vi "Serial Table Lookup.vi"(8 "error in (no error)":errorcluster, 9 "Target Serial#:":u32 caption="Serial#:" max=268435455, 10 "Data IN":T1={"Message"="", "Homed?"=FALSE, "NextState"=enum."Timeout", "G.Load"=0.0, "G.Position"=0.0, "Load#"=0, "[G.Loads]"=[], "[TotalLoads]"=[], "[Errors]"=[], "ZeroWait"=0, "Results"=[], "DwellWait"=FALSE, "Test Result"=FALSE, "[CondyleLoads]"=[], "[Max]"=[], "[Min]"=[], "Valid String?"=FALSE, "ScanTime"=timestamp(0 s since 1904-01-01), "ScannedString"="", "LabelDevID"=0, "MfgDate"=timestamp(0 s since 1904-01-01), "[EEPROM Cmds]"=[], "[CalData]"=[], "[A/Ds]"=[], "[A/Dmax]"=[], "[A/Dmin]"=[], "BattMax"=0.0, "BattMin"=0.0, "DwellTime"=2000, "PendingDeviceType"="", "Zero G.load"=0.0, "GAINC Value"="", "Programming Step"=enum."Load EEPROM", "Front Panel Program?"=FALSE, "Final Program?"=FALSE, "PCB Score"=100, "AssyScore"=100, "Pass/Fail #"="", "Result String"="", "Programming Mode"=enum."Initial Program", "Angle Test Step"=enum."Initialize", "Accel Values"=[], "Shutdown Counter"=0, "V1"=0, "V2"=0, "V3"=0, "V4"=0, "EEPROM Data"=[], "Counter"=0, "Page#"=0, "Timer"=timestamp(0 s since 1904-01-01), "Use Mark10?"=FALSE, "Eng-Result#"=0, "DUT Serial #"=0, "Scroll Message?"=FALSE, "Clear Message"=FALSE, "Batt Test Step "=enum."Initialize", "RXTX Window Found?"=FALSE, "Shutdown First Call?"=FALSE, "A2 Delay (msec)"=500, "Support Script"={"Script #"="", "Script Revision"="", "[OEMs]"=[], "[[DeviceTypes]]"=[], "[[DeviceTypesVals]]"=[], "[[List of Errors]]"=[], "Default GAINC"="", "[[ASICtrims]]"=[], "ID For Echo"="", "Condyle A CalFactor"=100, "Condyle B CalFactor"=100, "[OEMs Prefix]"=[], "Packet ID 18"="", "[[Force Table Load Test]]"=[], "[[Force Table AccurTest]]"=[]}, "Serial Table"={"Serial File Path"=path "", "[[Serial Lookup Table]]"=[], "Serial Device Info"=[], "Valid Serial?"=FALSE}, "Target Information"={"Target Brand"="", "Target DeviceType"="", "Target Serial#"=100, "Target Lot#"=0, "Target DevID"=0, "Target Channel"=5}, "Operator"="", "COM Port"="", "Config Path"=path "", "Tx Array"=[], "DUT Parameters"={"Channel"=0, "DeviceID"=0, "Script Rev"=0, "Month"=0, "Day"=0, "Year"=0, "Lot#"=0, "V1"=0, "V2"=0, "V3"=0, "V4"=0, "MFG"=0, "Cal FactorA 10"=0, "Cal FactorB 10  "=0, "Cal FactorA 16"=0, "Cal FactorB 16"=0, "ASICtrim"=[], "TmpChan"=0, "GAINC"="", "Brand"="", "Device"="", "Serial #"=0, "Batt310"=0, "Batt 280"=0}, "FTS Main?"=FALSE, "Loading"={"[Forces]"=[], "[Dwell]"=[], "Loading Step"=enum."Initialize Test"}, "Software Version"="", "Correction Factor"="", "Second Load Test"=FALSE, "Acc Loads"=[], "Mark10 Config"={"H2S%"=[80.0, 85.0, 90.0, 95.0, 100.0], "H2S Speed"=[12.0, 8.0, 6.0, 4.0, 2.0], "H to S"=2.0, "Home Speed"=1.0, "LoadWin"=0.0, "Load Speed"=0.0, "PID"={"Kp"=0.04, "Kd"=0.005001, "Ki"=2.9999999999999923e-05}}, "Channels"={"Transceiver Ch"=5, "Operating Ch"=5, "Start Ch"=0}, "Channel EEPROM"=[], "Load Notes"=[], "Engr Log?"=FALSE, "Time"=[], "Program Retry"=FALSE, "Operator Channel"="", "Target Channel "="", "New Data Program"=FALSE, "NFHU Pass?"=FALSE, "Cycle Number"=0, "Cal Cycle#"=0, "[Avg G.Loads] "=[], "[Avg A/Ds] "=[], "Cal Retry?"=FALSE, "[Total A/Ds]  "=[], "Cycle Num LA"=0, "LA Cycle# "=0, "Shim Num"=0, "Shim#  "=0, "Angle Test?"=FALSE} {"Mark10 Config"."PID"."Ki" min=0.0 max=200.0 format="%.6f"; "Mark10 Config"."PID"."Kd" min=0.0 max=200.0 format="%.6f"; "Mark10 Config"."PID"."Kp" min=0.0 max=200.0 format="%.6f"; "DUT Parameters"."ASICtrim" format="%02x"}) -> (0 "error out":errorcluster, 2 "Valid Serial":bool, 3 "State-machine Local Variables out":T1={"Message"="", "Homed?"=FALSE, "NextState"=enum."Timeout", "G.Load"=0.0, "G.Position"=0.0, "Load#"=0, "[G.Loads]"=[], "[TotalLoads]"=[], "[Errors]"=[], "ZeroWait"=0, "Results"=[], "DwellWait"=FALSE, "Test Result"=FALSE, "[CondyleLoads]"=[], "[Max]"=[], "[Min]"=[], "Valid String?"=FALSE, "ScanTime"=timestamp(0 s since 1904-01-01), "ScannedString"="", "LabelDevID"=0, "MfgDate"=timestamp(0 s since 1904-01-01), "[EEPROM Cmds]"=[], "[CalData]"=[], "[A/Ds]"=[], "[A/Dmax]"=[], "[A/Dmin]"=[], "BattMax"=0.0, "BattMin"=0.0, "DwellTime"=2000, "PendingDeviceType"="", "Zero G.load"=0.0, "GAINC Value"="", "Programming Step"=enum."Load EEPROM", "Front Panel Program?"=FALSE, "Final Program?"=FALSE, "PCB Score"=100, "AssyScore"=100, "Pass/Fail #"="", "Result String"="", "Programming Mode"=enum."Initial Program", "Angle Test Step"=enum."Initialize", "Accel Values"=[], "Shutdown Counter"=0, "V1"=0, "V2"=0, "V3"=0, "V4"=0, "EEPROM Data"=[], "Counter"=0, "Page#"=0, "Timer"=timestamp(0 s since 1904-01-01), "Use Mark10?"=FALSE, "Eng-Result#"=0, "DUT Serial #"=0, "Scroll Message?"=FALSE, "Clear Message"=FALSE, "Batt Test Step "=enum."Initialize", "RXTX Window Found?"=FALSE, "Shutdown First Call?"=FALSE, "A2 Delay (msec)"=500, "Support Script"={"Script #"="", "Script Revision"="", "[OEMs]"=[], "[[DeviceTypes]]"=[], "[[DeviceTypesVals]]"=[], "[[List of Errors]]"=[], "Default GAINC"="", "[[ASICtrims]]"=[], "ID For Echo"="", "Condyle A CalFactor"=100, "Condyle B CalFactor"=100, "[OEMs Prefix]"=[], "Packet ID 18"="", "[[Force Table Load Test]]"=[], "[[Force Table AccurTest]]"=[]}, "Serial Table"={"Serial File Path"=path "", "[[Serial Lookup Table]]"=[], "Serial Device Info"=[], "Valid Serial?"=FALSE}, "Target Information"={"Target Brand"="", "Target DeviceType"="", "Target Serial#"=100, "Target Lot#"=0, "Target DevID"=0, "Target Channel"=5}, "Operator"="", "COM Port"="", "Config Path"=path "", "Tx Array"=[], "DUT Parameters"={"Channel"=0, "DeviceID"=0, "Script Rev"=0, "Month"=0, "Day"=0, "Year"=0, "Lot#"=0, "V1"=0, "V2"=0, "V3"=0, "V4"=0, "MFG"=0, "Cal FactorA 10"=0, "Cal FactorB 10  "=0, "Cal FactorA 16"=0, "Cal FactorB 16"=0, "ASICtrim"=[], "TmpChan"=0, "GAINC"="", "Brand"="", "Device"="", "Serial #"=0, "Batt310"=0, "Batt 280"=0}, "FTS Main?"=FALSE, "Loading"={"[Forces]"=[], "[Dwell]"=[], "Loading Step"=enum."Initialize Test"}, "Software Version"="", "Correction Factor"="", "Second Load Test"=FALSE, "Acc Loads"=[], "Mark10 Config"={"H2S%"=[80.0, 85.0, 90.0, 95.0, 100.0], "H2S Speed"=[12.0, 8.0, 6.0, 4.0, 2.0], "H to S"=2.0, "Home Speed"=1.0, "LoadWin"=0.0, "Load Speed"=0.0, "PID"={"Kp"=0.04, "Kd"=0.005001, "Ki"=2.9999999999999923e-05}}, "Channels"={"Transceiver Ch"=5, "Operating Ch"=5, "Start Ch"=0}, "Channel EEPROM"=[], "Load Notes"=[], "Engr Log?"=FALSE, "Time"=[], "Program Retry"=FALSE, "Operator Channel"="", "Target Channel "="", "New Data Program"=FALSE, "NFHU Pass?"=FALSE, "Cycle Number"=0, "Cal Cycle#"=0, "[Avg G.Loads] "=[], "[Avg A/Ds] "=[], "Cal Retry?"=FALSE, "[Total A/Ds]  "=[], "Cycle Num LA"=0, "LA Cycle# "=0, "Shim Num"=0, "Shim#  "=0, "Angle Test?"=FALSE} {"Mark10 Config"."PID"."Ki" min=0.0 max=200.0 format="%.6f"; "Mark10 Config"."PID"."Kd" min=0.0 max=200.0 format="%.6f"; "Mark10 Config"."PID"."Kp" min=0.0 max=200.0 format="%.6f"; "DUT Parameters"."ASICtrim" format="%02x"})   [LabVIEW 2015]
uses:
  Controls/LocalVars.ctl
  Controls/Gen2 FT states.ctl
  Controls/Iniial Device Programming.ctl
  ProgramStageControl.ctl
  Controls/Batt Cap Steps.ctl
  Controls/Support Script.ctl
  Controls/Serial Table.ctl
  Controls/Device Information.ctl
  Controls/InfoPacket.ctl
  Controls/Loading.ctl
  Controls/Load Step.ctl
  Controls/Mark10 Config.ctl
  Controls/PID parameters.ctl
  Controls/Channels.ctl
panel:
  out "[[DeviceTypesVals]]":u16[][](array[numeric])
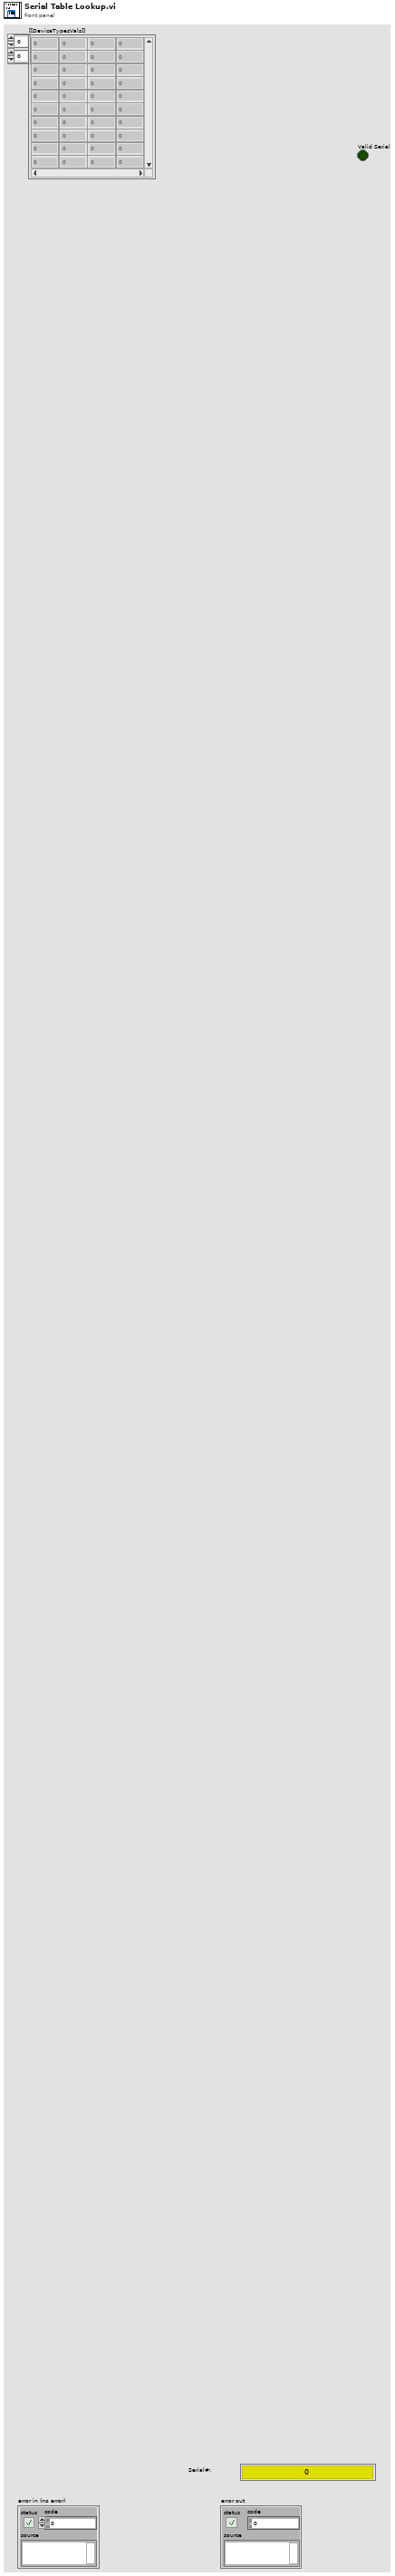
[diagram p1: front panel]
types:
  T1 = typedef "LocalVars.ctl" = cluster{"Message":string, "Homed?":bool, "NextState":T2, "G.Load":dbl, "G.Position":dbl, "Load#":i32, "[G.Loads]":dbl[], "[TotalLoads]":dbl[], "[Errors]":dbl[][], "ZeroWait":u32, "Results":dbl[], "DwellWait":bool, "Test Result":bool, "[CondyleLoads]":dbl[][], "[Max]":dbl[], "[Min]":dbl[], "Valid String?":bool, "ScanTime":timestamp, "ScannedString":string, "LabelDevID":u32, "MfgDate":timestamp, "[EEPROM Cmds]":u8[][], "[CalData]":u8[][], "[A/Ds]":dbl[][], "[A/Dmax]":dbl[], "[A/Dmin]":dbl[], "BattMax":dbl, "BattMin":dbl, "DwellTime":i32, "PendingDeviceType":string, "Zero G.load":dbl, "GAINC Value":string, "Programming Step":T3, "Front Panel Program?":bool, "Final Program?":bool, "PCB Score":i32, "AssyScore":i32, "Pass/Fail #":string, "Result String":string, "Programming Mode":T4, "Angle Test Step":enum16{"Initialize", "Get X", "Get Y", "Get Z", "Next Test"}, "Accel Values":dbl[][], "Shutdown Counter":u32, "V1":i32, "V2":i32, "V3":i32, "V4":i32, "EEPROM Data":i32[][], "Counter":i32, "Page#":i32, "Timer":timestamp, "Use Mark10?":bool, "Eng-Result#":u32, "DUT Serial #":i32, "Scroll Message?":bool, "Clear Message":bool, "Batt Test Step ":T5, "RXTX Window Found?":bool, "Shutdown First Call?":bool, "A2 Delay (msec)":i16, "Support Script":T6, "Serial Table":T7, "Target Information":T8, "Operator":string, "COM Port":string, "Config Path":path, "Tx Array":u8[], "DUT Parameters":T9, "FTS Main?":bool, "Loading":T10, "Software Version":string, "Correction Factor":string, "Second Load Test":bool, "Acc Loads":dbl[][], "Mark10 Config":T12, "Channels":T14, "Channel EEPROM":i32[][], "Load Notes":string[], "Engr Log?":bool, "Time":timestamp[], "Program Retry":bool, "Operator Channel":string, "Target Channel ":string, "New Data Program":bool, "NFHU Pass?":bool, "Cycle Number":i32, "Cal Cycle#":i32, "[Avg G.Loads] ":dbl[], "[Avg A/Ds] ":dbl[][], "Cal Retry?":bool, "[Total A/Ds]  ":dbl[][], "Cycle Num LA":i32, "LA Cycle# ":i32, "Shim Num":i32, "Shim#  ":i32, "Angle Test?":bool}
  T2 = typedef "Gen2 FT states.ctl" = enum16{"---------SETUP-------", "Initialization", "Read Support Data", "Initialize Mark-10", "Initialize Transceiver", "------UTILITIES------", "Change DUT Channel", "Find RxTx Window", "Reset Device", "Scan Channels", "Read Serial Lookup", "Shutdown Device", "ESTOP", "--------USER---------", "Timeout", "-----PROGRAM-----", "Program Device", "------MARK10--------", "Go Home", "MoveUp", "MoveDown", "Goto Load", "Goto Position", "Stop Motor", "---------TESTS--------", "Start Test", "Angle Test", "Load Test", "Load Accuracy Test", "Battery Test", "------RESULTS-------", "End Test", "Display Result", "--------EXIT--------", "Exit"}
  T3 = typedef "Iniial Device Programming.ctl" = enum16{"Load EEPROM", "Send First A1", "Send EEPROM", "Send A1", "Check EEPROM Echo", "Verify transmission", "Programming Successful", "Programming Failed"}
  T4 = typedef "ProgramStageControl.ctl" = enum16{"Initial Program", "GainC", "Scales"}
  T5 = typedef "Batt Cap Steps.ctl" = enum16{"Initialize", "Collect 2.8 Volts", "Collect 3.1 Volts", "Check Results"}
  T6 = typedef "Support Script.ctl" = cluster{"Script #":string, "Script Revision":string, "[OEMs]":string[], "[[DeviceTypes]]":string[][], "[[DeviceTypesVals]]":u16[][], "[[List of Errors]]":string[][], "Default GAINC":string, "[[ASICtrims]]":u8[][], "ID For Echo":string, "Condyle A CalFactor":i32, "Condyle B CalFactor":i32, "[OEMs Prefix]":string[], "Packet ID 18":string, "[[Force Table Load Test]]":dbl[][], "[[Force Table AccurTest]]":dbl[][]}
  T7 = typedef "Serial Table.ctl" = cluster{"Serial File Path":path, "[[Serial Lookup Table]]":string[][], "Serial Device Info":string[], "Valid Serial?":bool}
  T8 = typedef "Device Information.ctl" = cluster{"Target Brand":string, "Target DeviceType":string, "Target Serial#":i32, "Target Lot#":u32, "Target DevID":u32, "Target Channel":u8}
  T9 = typedef "InfoPacket.ctl" = cluster{"Channel":u8, "DeviceID":u32, "Script Rev":u8, "Month":u8, "Day":u8, "Year":u8, "Lot#":u32, "V1":u16, "V2":u16, "V3":u16, "V4":u16, "MFG":u8, "Cal FactorA 10":u8, "Cal FactorB 10  ":u8, "Cal FactorA 16":u8, "Cal FactorB 16":u8, "ASICtrim":u8[], "TmpChan":u8, "GAINC":string, "Brand":string, "Device":string, "Serial #":u64, "Batt310":u16, "Batt 280":u16}
  T10 = typedef "Loading.ctl" = cluster{"[Forces]":dbl[], "[Dwell]":dbl[], "Loading Step":T11}
  T11 = typedef "Load Step.ctl" = enum16{"Initialize Test", "Go Home", "Detect Dev Surface", "Wait to zero Device", "Zero Device", "Do Test", "Test Result"}
  T12 = typedef "Mark10 Config.ctl" = cluster{"H2S%":dbl[], "H2S Speed":dbl[], "H to S":dbl, "Home Speed":dbl, "LoadWin":dbl, "Load Speed":dbl, "PID":T13}
  T13 = typedef "PID parameters.ctl" = cluster{"Kp":dbl, "Kd":dbl, "Ki":dbl}
  T14 = typedef "Channels.ctl" = cluster{"Transceiver Ch":u8, "Operating Ch":u8, "Start Ch":u8}
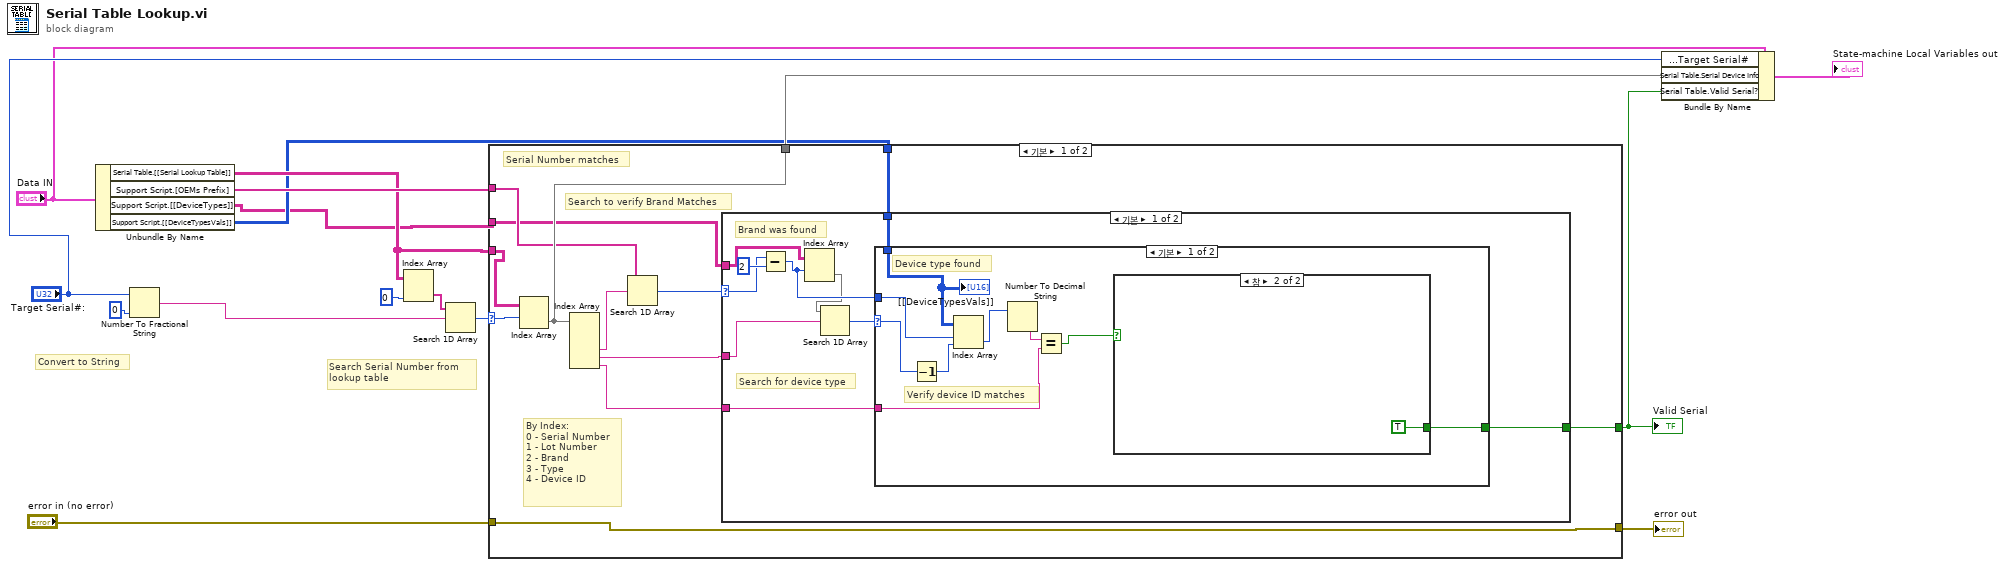
[diagram p0: block diagram]
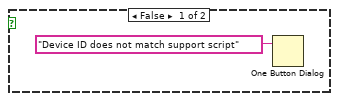
[diagram p2: hidden frame]
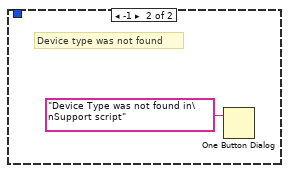
[diagram p3: hidden frame]
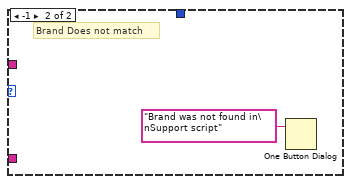
[diagram p4: hidden frame]
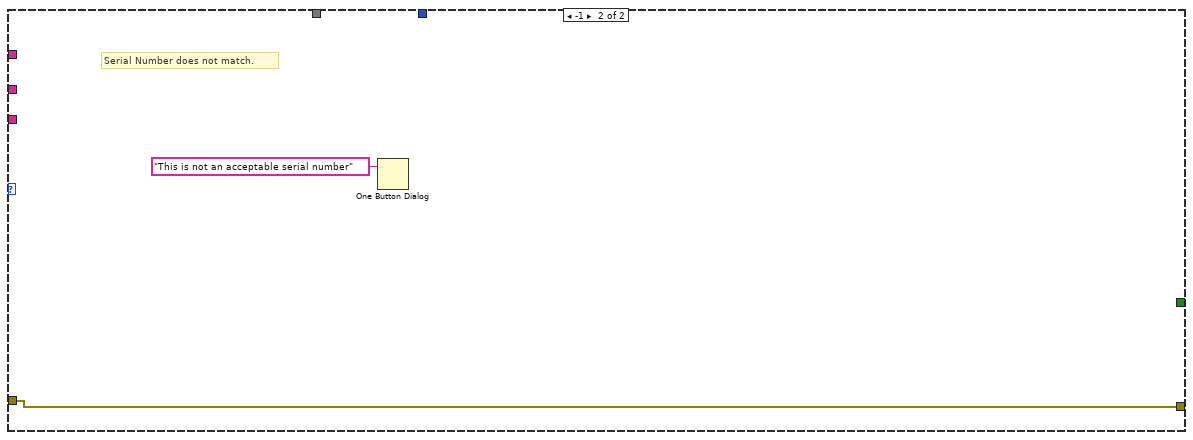
[diagram p5: hidden frame]
diagram:
  # "Search Serial Number from \nlookup table"
  # "Convert to String"
  n1 = Unbundle By Name("Data IN") -> ("Serial Table.[[Serial Lookup Table]]"=w6:string[][], "Support Script.[OEMs Prefix]"=w7:string[], "Support Script.[[DeviceTypes]]"=w1:string[][], "Support Script.[[DeviceTypesVals]]"=w5:u16[][])
  n2 = Number To Fractional String(number="Target Serial#:", precision (6)=i16 0) -> (F-format string=w13:string)  [unwired: 2 in]
  n3 = Index Array(array=w6, index (col)=0 ("disabled index (col)")) -> (element=w12:string[])  [unwired: 1 in]
  n4 = Search 1D Array(1D array=w12, element=w13) -> (index of element=w14:i32)  [unwired: 1 in]
  n5 = case shown="기본" w14 {
    selector: w14 -> [w28 _]
    tunnel: [w27 _] -> w8
    tunnel: w7 -> [w26 _]
    tunnel: w6 -> [w25 _]
    tunnel: w1 -> [w22 _]
    tunnel: w5 -> [w20 _]
    tunnel: [w18 _] -> w2
    tunnel: "error in (no error)" -> [w17 w52]
    tunnel: [w17 w52] -> w3
    frame Default {
      # "Search to verify Brand Matches"
      # "Serial Number matches"
      # "By Index:\n0 - Serial Number\n1 - Lot Number\n2 - Brand\n3 - Type\n4 - Device ID"
      n6 = Index Array(array=w25, index (row)=w28) -> (element=w27:string[])  [unwired: 1 in]
      n7 = Index Array(array=w27) -> (element #3=w24:string, element #4=w21:string, element #5=w19:string)  [unwired: 5 in, 2 out]
      n8 = Search 1D Array(1D array=w26, element=w24) -> (index of element=w23:i32)  [unwired: 1 in]
      n9 = case shown="기본" w23 {
        selector: w23 -> [w31 _]
        tunnel: w22 -> [w32 _]
        tunnel: w21 -> [w37 _]
        tunnel: w20 -> [w36 _]
        tunnel: w19 -> [w35 _]
        tunnel: [w34 _] -> w18
        frame Default {
          # "Search for device type"
          # "Brand was found"
          n10 = Subtract(x=w31, y=2) -> (x-y=w30:i32)
          n11 = Index Array(array=w32, index (row)=w30) -> (element=w29:string[])  [unwired: 1 in]
          n12 = Search 1D Array(1D array=w29, element=w37) -> (index of element=w38:i32)  [unwired: 1 in]
          n13 = case shown="기본" w38 {
            selector: w38 -> [w47 _]
            tunnel: w36 -> [w45 _]
            tunnel: w35 -> [w42 _]
            tunnel: [w40 _] -> w34
            tunnel: w30 -> [w39 _]
            frame Default {
              # "Verify device ID matches"
              # "Device type found"
              n14 = Decrement(x=w47) -> (x-1=w46:i32)
              n15 = Index Array(array=w45, index (row)=w39, index (col)=w46) -> (element=w44:u16)
              n16 = Number To Decimal String(number=w44) -> (decimal integer string=w43:string)  [unwired: 1 in]
              n17 = Equal?(x=w43, y=w42) -> (x = y?=w41:bool)
              n18 = case shown="참" w41 {
                tunnel: [_ TRUE] -> w40
                frame False {
                  n19 = One Button Dialog(message="Device ID does not match support script") -> ()  [unwired: 1 in, 1 out]
                }
                frame True {
                }
              }
              "[[DeviceTypesVals]]" <- w45
            }
            frame -1 {
              # "Device type was not found"
              n20 = One Button Dialog(message="Device Type was not found in\nSupport script") -> ()  [unwired: 1 in, 1 out]
            }
          }
        }
        frame -1 {
          # "Brand Does not match"
          n21 = One Button Dialog(message="Brand was not found in\nSupport script") -> ()  [unwired: 1 in, 1 out]
        }
      }
    }
    frame -1 {
      # "Serial Number does not match."
      n22 = One Button Dialog(message="This is not an acceptable serial number") -> ()  [unwired: 1 in, 1 out]
    }
  }
  "error out" <- w3
  "Valid Serial" <- w2
  n23 = Bundle By Name(cluster="Data IN", "Target Information.Target Serial#"="Target Serial#:", "Serial Table.Serial Device Info"=w8, "Serial Table.Valid Serial?"=w2) -> (→"State-machine Local Variables out":T1)
